vi "Set Frequency.vi"(8 "error in (no error)":errorcluster, 10 "Frequency (1000Hz)":dbl=1000.0, 11 "PWM in":refnum<class "LINX-PCA9685 PWM.lvclass">) -> (0 "error out":errorcluster, 3 "PWM out":refnum<class "LINX-PCA9685 PWM.lvclass">)   [LabVIEW 2020, in "LINX-PCA9685 PWM.lvclass"]
uses:
  LINX-PCA9685 PWM.lvclass
  LINX I2C/LINX I2C.lvclass
panel:
  out "Prescale Value":dbl
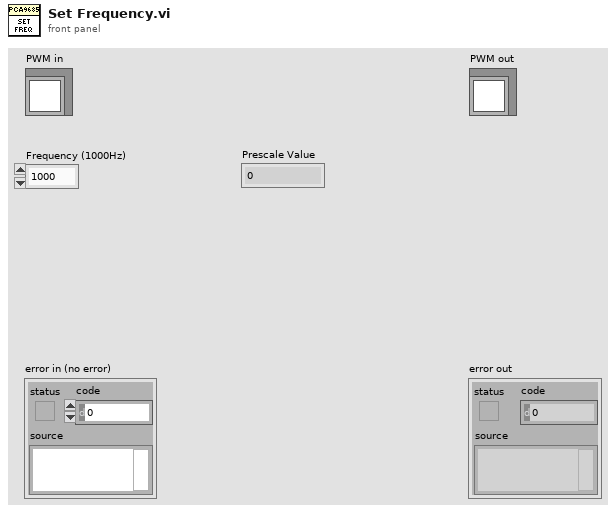
[diagram p1: front panel]
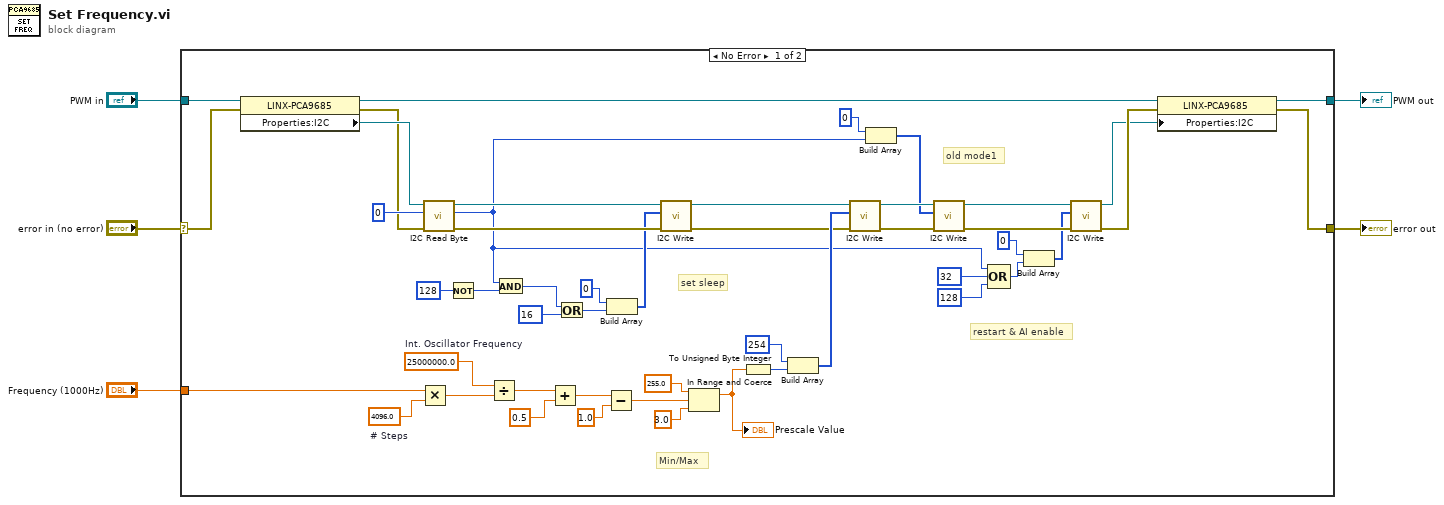
[diagram p0: block diagram]
diagram:
  n1 = case shown="No Error" "error in (no error)" {
    selector: "error in (no error)" -> [w13 w55]
    tunnel: [w7 w55] -> w4
    tunnel: [w6 w54] -> w2
    tunnel: "PWM in" -> [w14 w54]
    tunnel: "Frequency (1000Hz)" -> [w53 _]
    frame No Error {
      w52 = 4096.0  # # Steps
      w51 = 25000000.0  # Int. Oscillator Frequency
      # "set sleep"
      # "old mode1"
      # "restart & AI enable"
      # "Min/Max"
      n2 = property class="LINX-PCA9685"(reference=w14, error in=w13) -> (reference out=w11:refnum<class "LINX-PCA9685 PWM.lvclass">, error out=w10:errorcluster, "Properties:I2C"=w12:refnum<class "LINX I2C.lvclass">)
      n3 = Multiply(x=w53, y=w52) -> (x*y=w50:dbl)
      n4 = call-dynamic "I2C Read Byte.vi"("error in (no error)"=w10, "Address"=u8 0, "LINX I2C in"=w12) -> ("error out"=w33:errorcluster, "Byte Read"=w20:u8, "LINX I2C out"=w30:refnum<class "LINX I2C.lvclass">)  [unwired: 6 in]
      n5 = Not(x=u8 128) -> (.not. x?=w36:u8)
      n6 = Divide(x=w51, y=w50) -> (x/y=w49:dbl)
      n7 = And(x=w20, y=w36) -> (x .and. y?=w35:u8)
      n8 = Add(x=w49, y=0.5 ("x")) -> (x+y=w47:dbl)
      n9 = Or(x=w35, y=u8 16) -> (x .or. y?=w28:u8)
      n10 = Subtract(x=w47, y=1.0) -> (x-y=w45:dbl)
      n11 = Build Array(u8 0 ("Address"), w28) -> (w27:u8[])
      n12 = call "I2C Write.vi"("error in (no error)"=w33, "Bytes to Write"=w27, "LINX I2C in"=w30) -> ("error out"=w32:errorcluster, "LINX I2C out"=w31:refnum<class "LINX I2C.lvclass">)  [unwired: 7 in]
      n13 = In Range and Coerce(upper limit=255.0, x=w45, lower limit=3.0) -> (coerced(x)=w42:dbl)  [unwired: 1 out]
      "Prescale Value" <- w42
      n14 = To Unsigned Byte Integer(number=w42) -> (unsigned 8bit integer=w41:u8)
      n15 = Build Array(u8 254 ("unsigned 8bit integer"), w41) -> (w40:u8[])
      n16 = call "I2C Write.vi"("error in (no error)"=w32, "Bytes to Write"=w40, "LINX I2C in"=w31) -> ("error out"=w26:errorcluster, "LINX I2C out"=w25:refnum<class "LINX I2C.lvclass">)  [unwired: 7 in]
      n17 = Build Array(u8 0 ("Address"), w20) -> (w23:u8[])
      n18 = call "I2C Write.vi"("error in (no error)"=w26, "Bytes to Write"=w23, "LINX I2C in"=w25) -> ("error out"=w21:errorcluster, "LINX I2C out"=w22:refnum<class "LINX I2C.lvclass">)  [unwired: 7 in]
      n19 = Compound Arithmetic op=OR(w20, u8 32, u8 128) -> (w16:u8)
      n20 = Build Array(u8 0 ("Address"), w16) -> (w15:u8[])
      n21 = call "I2C Write.vi"("error in (no error)"=w21, "Bytes to Write"=w15, "LINX I2C in"=w22) -> ("error out"=w9:errorcluster, "LINX I2C out"=w8:refnum<class "LINX I2C.lvclass">)  [unwired: 7 in]
      n22 = property class="LINX-PCA9685"(reference=w11, error in=w9, "Properties:I2C"=w8) -> (reference out=w6:refnum<class "LINX-PCA9685 PWM.lvclass">, error out=w7:errorcluster)
    }
    frame Error {
    }
  }
  "error out" <- w4
  "PWM out" <- w2
